vi "Auto Scorer.vi"() -> ()   [LabVIEW 2024, in "Wordle Scorer.lvlib"]
uses:
  Wordle Scorer.lvlib
  Scorer State.ctl
  Scoring Result.ctl
panel:
  out "tskill output":string
  in  "Poll Now":bool
  out "Response":string
  out "Scoring Result":T1
  out "Run Time":dbl format="%<%M:%S%1u>t"
  out "Run Start":timestamp
  out "VI Refnum":refnum<vi>
  out "App Ref":refnum<vi>
  out "Zip":path
  out "Upload Error":errorcluster
  out "Score Error":errorcluster
  out "Download Error":errorcluster
  out "Poll Error":errorcluster
  out "Last Poll":timestamp format="%<%Y-%m-%d %H:%M:%S>T"
  out "State":T2
  out "Previous Submission":i32
  out "Current Submission":i32
  out "Time to next poll":dbl format="%#.0f"
  in  "Poll Period":dbl=60.0
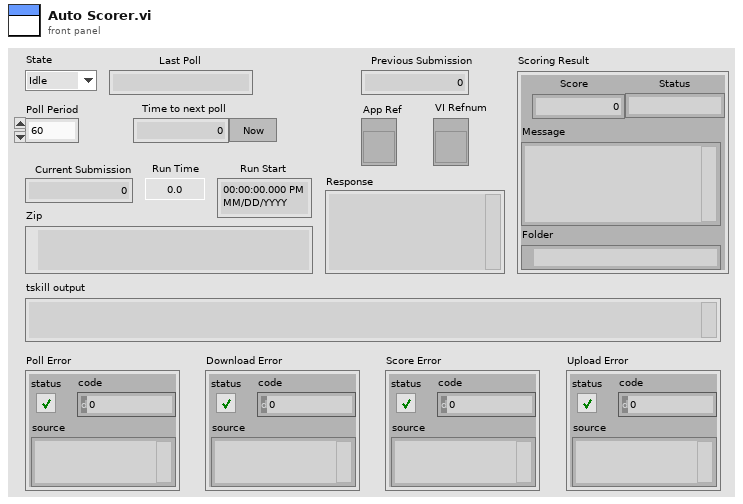
[diagram p1: front panel]
types:
  T1 = typedef "Wordle Scorer.lvlib/Scoring Result.ctl" = cluster{"Score":dbl, "Status":string, "Message":string, "Folder":path}
  T2 = typedef "Wordle Scorer.lvlib/Scorer State.ctl" = enum16{"Idle", "Poll", "Run", "Upload", "Error", "Timeout"}
  T3 = enum32{"Bad", "Idle", "Run top level", "Running"}
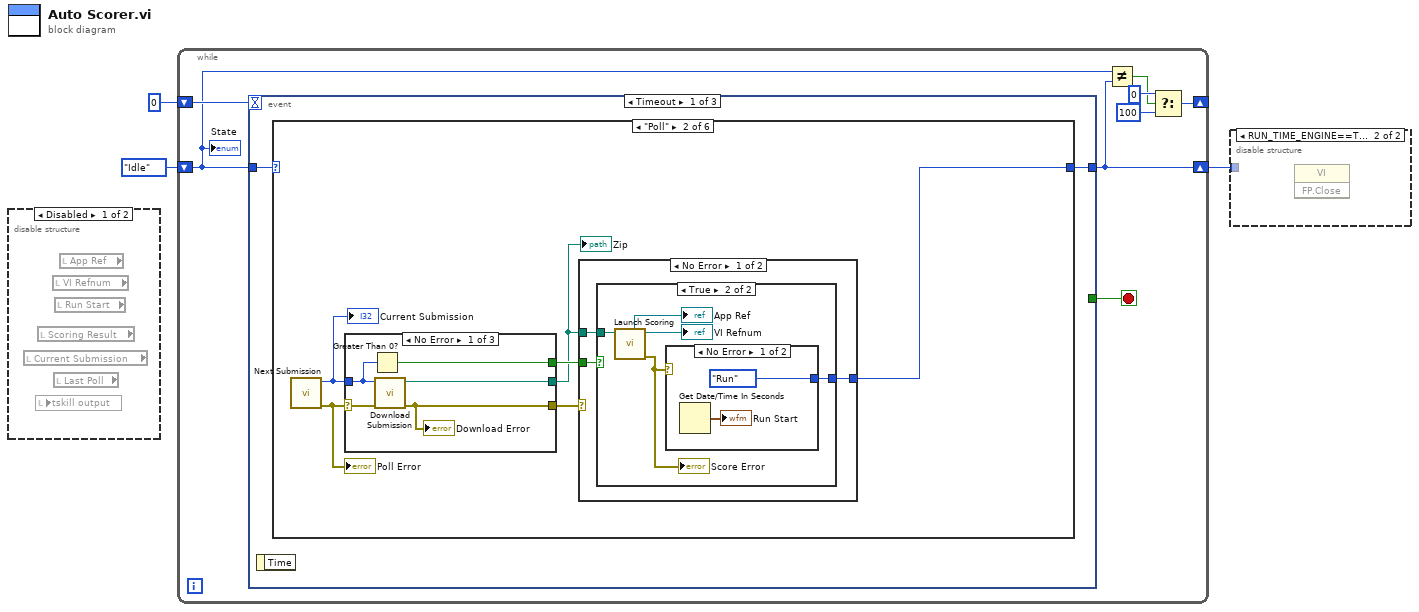
[diagram p0: block diagram]
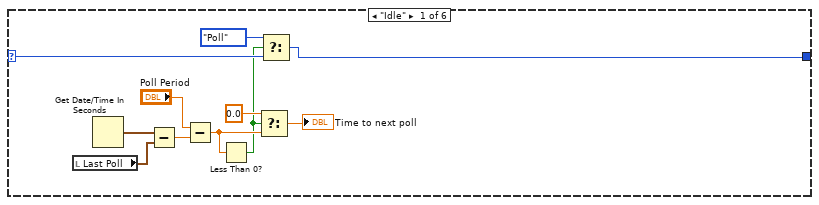
[diagram p4: hidden frame]
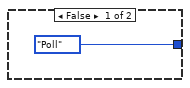
[diagram p5: hidden frame]
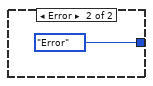
[diagram p6: hidden frame]
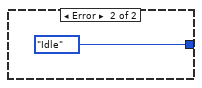
[diagram p7: hidden frame]
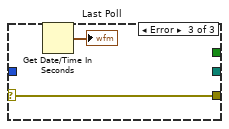
[diagram p9: hidden frame]
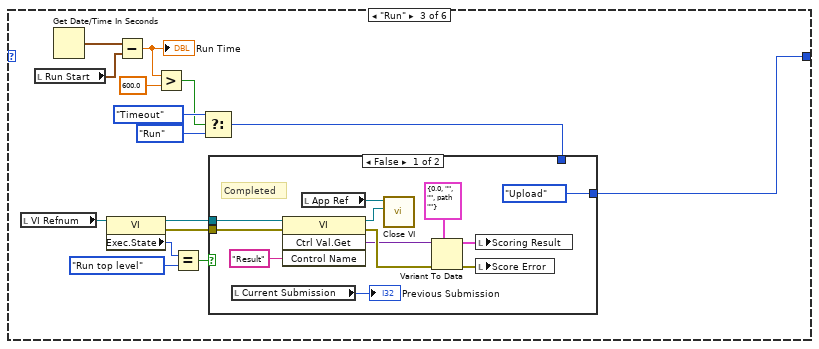
[diagram p10: hidden frame]
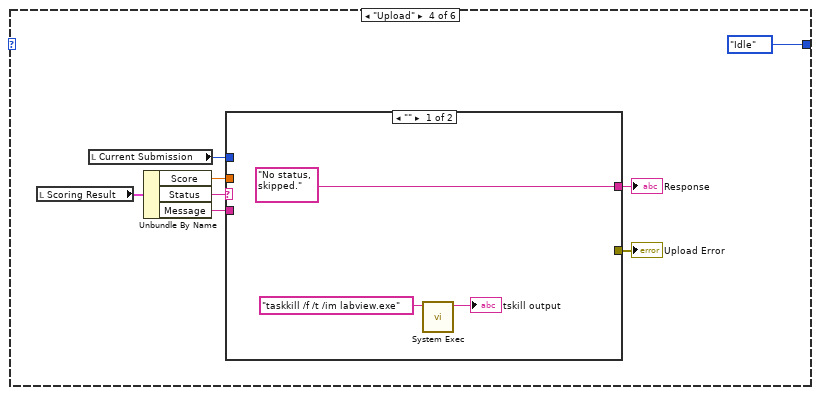
[diagram p12: hidden frame]
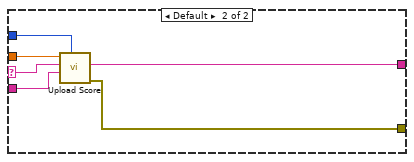
[diagram p13: hidden frame]
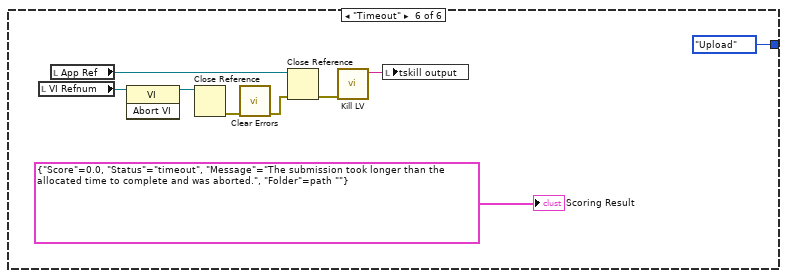
[diagram p15: hidden frame]
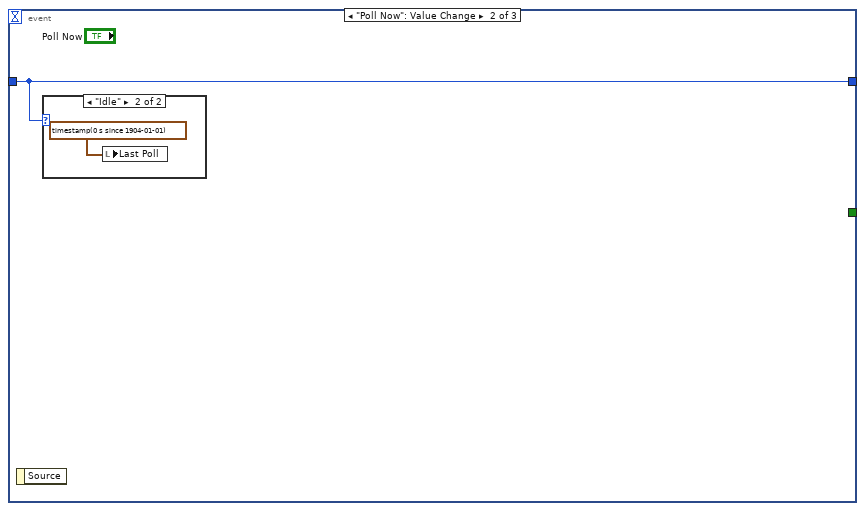
[diagram p16: hidden frame]
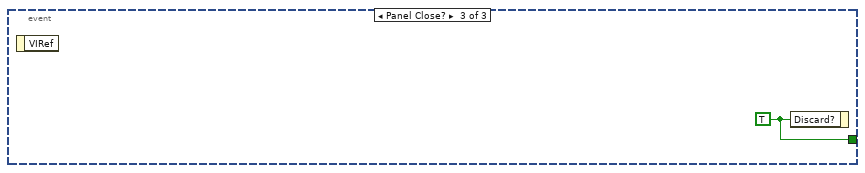
[diagram p18: hidden frame]
diagram:
  n1 = disable-structure shown="Disabled" {
    frame Disabled {
      n2 = local read "Current Submission"() -> ()  [unwired: 1 out]
      n3 = local read "tskill output"() -> ()  [unwired: 1 in]
      n4 = local read "Scoring Result"() -> ()  [unwired: 1 out]
      n5 = local read "VI Refnum"() -> ()  [unwired: 1 out]
      n6 = local read "Last Poll"() -> ()  [unwired: 1 out]
      n7 = local read "Run Start"() -> ()  [unwired: 1 out]
      n8 = local read "App Ref"() -> ()  [unwired: 1 out]
    }
    frame Enabled {
    }
  }
  n9 = while {
    shift-right: [w10] -> w1
    shift-left: Scorer_State."Idle" ("Scorer State") -> [w9]
    shift-right: [w7] -> _
    shift-left: 0 -> [w11]
    stop <- w4 stop-if-true
    n10 = event shown="[0] Timeout" {
      selector: _ -> [_ _ _]
      dyn-events: _ -> [_ _ _]
      timeout: w11 -> [_ _ _]
      tunnel: w9 -> [w13 w107 _]
      tunnel: [w12 w107 _] -> w10
      tunnel: [_ _ w109] -> w4
      event Timeout {
        n11 = event-data() -> ()  [unwired: 1 in, 1 out]
        n12 = case shown="\"Poll\"" w13 {
          selector: w13 -> [w17 _ _ _ w97 _]
          tunnel: [w14 w27 w60 Scorer_State."Idle" ("Scorer State") w97 Scorer_State."Upload" ("Scorer State")] -> w12
          frame "Idle" {
            n13 = local read "Last Poll"() -> (w23:timestamp)
            n14 = Get Date/Time In Seconds() -> (seconds since 1Jan1904=w24:timestamp)
            n15 = Subtract(x=w24, y=w23) -> (x-y=w22:dbl)
            n16 = Subtract(x="Poll Period", y=w22) -> (x-y=w20:dbl)
            n17 = Less Than 0?(x=w20) -> (x < 0?=w16:bool)
            n18 = Select(t=0.0, s=w16, f=w20) -> (s? t:f=→"Time to next poll":dbl)
            n19 = Select(t=Scorer_State."Poll", s=w16, f=w17) -> (s? t:f=w14:T2)
          }
          frame "Poll" {
            n20 = call "Next Submission.vi"() -> ("error out"=w29:errorcluster, "submission"=w25:i32)  [unwired: 9 in, 1 out]
            "Poll Error" <- w29
            "Current Submission" <- w25
            n21 = case shown="No Error" w29 {
              selector: w29 -> [w47 w49 w50]
              tunnel: w25 -> [w48 _ _]
              tunnel: [w46 _ _] -> w26
              tunnel: [w45 w49 w50] -> w30
              tunnel: [w44 _ _] -> w28
              frame No Error {
                n22 = Greater Than 0?(x=w48) -> (x > 0?=w44:bool)
                n23 = call "Download Submission.vi"("error in (no error)"=w47, "submission"=w48) -> ("error out"=w45:errorcluster, "Zip Path"=w46:path)  [unwired: 7 in, 1 out]
                "Download Error" <- w45
              }
              frame Default {
              }
              frame Error {
                # "No submissions"
                n24 = Get Date/Time In Seconds() -> (seconds since 1Jan1904=→"Last Poll":timestamp)
              }
            }
            "Zip" <- w26
            n25 = case shown="No Error" w30 {
              tunnel: w28 -> [w33 _]
              tunnel: [w32 Scorer_State."Idle" ("Scorer State")] -> w27
              tunnel: w26 -> [w31 _]
              frame No Error {
                n26 = case shown="True" w33 {
                  tunnel: [Scorer_State."Poll" ("Scorer State") w38] -> w32
                  tunnel: w31 -> [_ w35]
                  frame False {
                  }
                  frame True {
                    n27 = call "Launch Scoring.vi"("Zip"=w35) -> ("error out"=w39:errorcluster, "VI Refnum"=→"VI Refnum":refnum<vi>, "App Ref"=→"App Ref":refnum<vi>)  [unwired: 8 in]
                    "Score Error" <- w39
                    n28 = case shown="No Error" w39 {
                      tunnel: [Scorer_State."Run" ("Scorer State") Scorer_State."Error" ("Scorer State")] -> w38
                      frame No Error {
                        n29 = Get Date/Time In Seconds() -> (seconds since 1Jan1904=→"Run Start":timestamp)
                      }
                      frame Error {
                      }
                    }
                  }
                }
              }
              frame Error {
              }
            }
          }
          frame "Run" {
            n30 = local read "VI Refnum"() -> (w66:refnum<vi>)
            n31 = local read "Run Start"() -> (w62:timestamp)
            n32 = Get Date/Time In Seconds() -> (seconds since 1Jan1904=w63:timestamp)
            n33 = property class="VI"(reference=w66) -> (reference out=w53:refnum<vi>, error out=w52:errorcluster, "Exec.State"=w65:T3)  [unwired: 1 in]
            n34 = Subtract(x=w63, y=w62) -> (x-y=w59:dbl)
            "Run Time" <- w59
            n35 = Greater?(x=w59, y=600.0) -> (0:w55:bool)
            n36 = Equal?(x=w65, y=T3."Run top level") -> (x = y?=w61:bool)
            n37 = Select(t=Scorer_State."Timeout" ("Scorer State"), s=w55, f=Scorer_State."Run" ("Scorer State")) -> (s? t:f=w54:T2)
            n38 = case shown="False" w61 {
              tunnel: [Scorer_State."Upload" ("Scorer State") w79] -> w60
              tunnel: w54 -> [_ w79]
              tunnel: w53 -> [w77 _]
              tunnel: w52 -> [w74 _]
              frame False {
                # "Completed"
                n39 = local read "Current Submission"() -> (→"Previous Submission":i32)
                n40 = invoke class="VI" method="Ctrl Val.Get"(reference=w77, error in=w74, "Control Name"="Result") -> (reference out=w68:refnum<vi>, error out=w78:errorcluster, "Get Control Value Variant"=w75:variant)  [unwired: 1 in, 1 out]
                n41 = local read "App Ref"() -> (w67:refnum<vi>)
                n42 = call "Close VI.vi"("VI Refnum"=w68, "App Ref"=w67) -> ()  [unwired: 10 in]
                n43 = Variant To Data(error in=w78, type=T1 {"Score"=0.0, "Status"="", "Message"="", "Folder"=path ""} ("Scoring Result"), Variant=w75) -> (data=w72:T1, error out=w71:errorcluster)
                n44 = local write "Scoring Result"(w72) -> ()
                n45 = local write "Score Error"(w71) -> ()
              }
              frame True {
                # "Still running"
              }
            }
          }
          frame "Upload" {
            n46 = local read "Scoring Result"() -> (w86:T1)
            n47 = local read "Current Submission"() -> (w84:i32)
            n48 = Unbundle By Name(w86) -> ("Score"=w85:dbl, "Status"=w83:string, "Message"=w82:string)
            n49 = case shown="\"\"" w83 {
              selector: w83 -> [_ w94]
              tunnel: w85 -> [_ w96]
              tunnel: w84 -> [_ w95]
              tunnel: w82 -> [_ w93]
              tunnel: [_ w92] -> w81
              tunnel: ["No status, skipped." ("Response") w91] -> w80
              frame "" {
                n50 = call <vilib>:"System Exec.vi"("command line"="taskkill /f /t /im labview.exe") -> ("standard output"=→"tskill output":string)  [unwired: 7 in, 3 out]
              }
              frame Default {
                n51 = call "Upload Score.vi"("submission"=w95, "result"=w93, "status"=w94, "Run Time"=w96) -> ("error out"=w92:errorcluster, "Response"=w91:string)  [unwired: 5 in, 1 out]
              }
            }
            "Upload Error" <- w81
            "Response" <- w80
          }
          frame "Error" {
            # "Whoops! Time to be saved!"
          }
          frame "Timeout" {
            n52 = local read "VI Refnum"() -> (w104:refnum<vi>)
            n53 = local read "App Ref"() -> (w100:refnum<vi>)
            n54 = invoke class="VI" method="Abort VI"(reference=w104) -> (reference out=w103:refnum<vi>)  [unwired: 2 in, 2 out]
            n55 = Close Reference(reference=w103) -> (error out=w102:errorcluster)  [unwired: 1 in]
            n56 = call <vilib>:"Clear Errors.vi"("error in (no error)"=w102) -> ("error out"=w101:errorcluster)  [unwired: 5 in, 1 out]
            n57 = Close Reference(reference=w100, error in (no error)=w101) -> (error out=w99:errorcluster)
            n58 = call "Kill LV.vi"("error in (no error)"=w99) -> ("Output"=w98:string)  [unwired: 9 in, 1 out]
            n59 = local write "tskill output"(w98) -> ()
            "Scoring Result" <- T1 {"Score"=0.0, "Status"="timeout", "Message"="The submission took longer than the allocated time to complete and was aborted.", "Folder"=path ""} ("Scoring Result")
          }
        }
      }
      event "Poll Now": Value Change {
        n60 = event-data() -> ()  [unwired: 1 in, 1 out]
        n61 = case shown="\"Idle\"" w107 {
          frame Default {
          }
          frame "Idle" {
            n62 = local write "Last Poll"(timestamp(0 s since 1904-01-01) ("Last Poll")) -> ()
          }
        }
      }
      event Panel Close? {
        w109 = TRUE ("Discard?")
        n63 = event-data() -> ()  [unwired: 1 in, 1 out]
        n64 = event-data("Discard?"=w109) -> ()  [unwired: 1 in, 1 out]
      }
    }
    n65 = Not Equal?(x=w9, y=w10) -> (x != y?=w5:bool)
    n66 = Select(t=0, s=w5, f=100) -> (s? t:f=w7:i32)
    "State" <- w9
  }
  n67 = disable-structure shown="RUN_TIME_ENGINE==True" {
    disable-tunnel: w1 -> [_ _]
    frame condition #0 (active) {
    }
    frame condition #1 {
      n68 = invoke class="VI" method="FP.Close"() -> ()  [unwired: 3 in, 3 out]
    }
  }
